vi "getCamRamAllocation.vi"(0 "Camera in":refnum<class "Camera.lvclass">, 11 "error in (no error)":errorcluster) -> (4 "Camera out":refnum<class "Camera.lvclass">, 6 "percents":u32[](array[numeric]), 15 "error out":errorcluster)   [LabVIEW 2019, in "Camera.lvclass"]
doc: "Returns the size of each CamRam segment as a percent of the total CamRAM size. Output is an array of percentages, one per segment. Returns an error if camera does not have internal memory."
uses:
  Camera.lvclass
  Camera.lvclass/Camera.ctl
  pco.sdk/StorageControl/StorageControl.lvlib
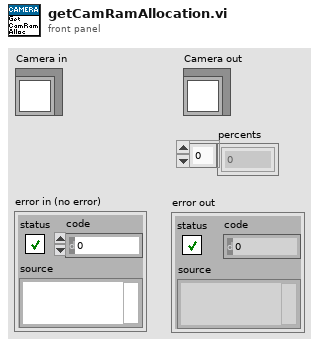
[diagram p1: front panel]
types:
  T1 = cluster{"dwRamSize":u32, "wPageSize":u16, "dwRamSegSize":u32[], "wActSeg":u16}
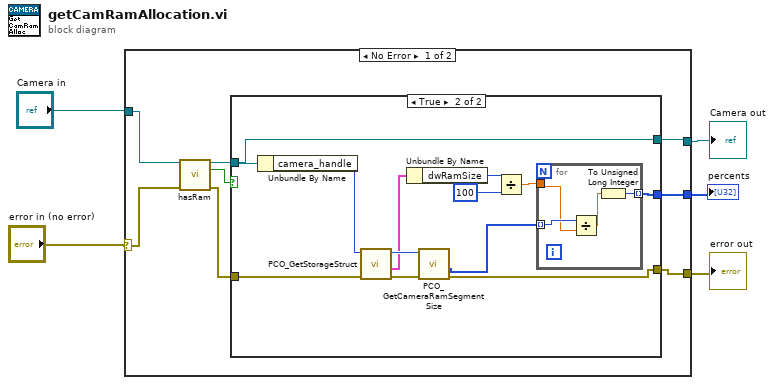
[diagram p0: block diagram]
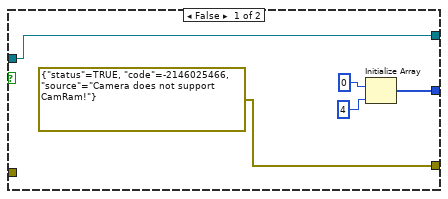
[diagram p2: hidden frame]
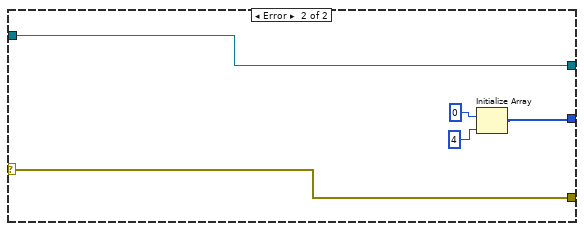
[diagram p3: hidden frame]
diagram:
  n1 = case shown="No Error" "error in (no error)" {
    selector: "error in (no error)" -> [w10 w39]
    tunnel: [w7 w39] -> w3
    tunnel: [w8 w38] -> w4
    tunnel: "Camera in" -> [w9 w38]
    tunnel: [w6 w35] -> w1
    frame No Error {
      n2 = call-dynamic "hasRam.vi"("Camera in"=w9, "error in (no error)"=w10) -> ("Camera out"=w13:refnum<class "Camera.lvclass">, "hasRam"=w12:bool, "error out"=w11:errorcluster)  [unwired: 11 in]
      n3 = case shown="True" w12 {
        tunnel: w11 -> [_ w30]
        tunnel: w13 -> [w17 w28]
        tunnel: [errorcluster {"status"=TRUE, "code"=-2146025466, "source"="Camera does not support CamRam!"} ("error constant") w19] -> w7
        tunnel: [w17 w28] -> w8
        tunnel: [w14 w20] -> w6
        frame False {
          n4 = Initialize Array(u32 0 ("dwRamSegSize"), 4 ("dimension size")) -> (w14:u32[])
        }
        frame True {
          n5 = Unbundle By Name(w28) -> ("camera_handle"=w29:u64)
          n6 = call "PCO_GetStorageStruct.vi"("error in (no error)"=w30, "ph"=w29) -> ("error out"=w26:errorcluster, "strStorage"=w24:T1, "ph out"=w27:u64)  [unwired: 6 in, 1 out]
          n7 = Unbundle By Name(w24) -> ("dwRamSize"=w23:u32)
          n8 = call "PCO_GetCameraRamSegmentSize.vi"("error in (no error)"=w26, "ph"=w27) -> ("error out"=w19:errorcluster, "dwRamSegSize"=w25:u32[])  [unwired: 6 in, 2 out]
          n9 = Divide(x=w23, y=u32 100) -> (x/y=w21:dbl)
          n10 = for {
            tunnel: w25 -> [w34] mode=indexing
            tunnel: w21 -> [w33]
            tunnel: [w31] -> w20 mode=indexing
            n11 = Divide(x=w34, y=w33) -> (x/y=w32:dbl)
            n12 = To Unsigned Long Integer(number=w32) -> (unsigned 32bit integer=w31:u32)
          }
        }
      }
    }
    frame Error {
      n13 = Initialize Array(u32 0 ("dwRamSegSize"), 4 ("dimension size")) -> (w35:u32[])
    }
  }
  "error out" <- w3
  "Camera out" <- w4
  "percents" <- w1
